vi "用户注册.vi"(8 "错误输入（无错误）":errorcluster, 11 "excel路径":path) -> (0 "错误输出":errorcluster)   [LabVIEW 2014]
panel:
  in  "取消注册":bool
  in  "注册":bool
  in  "入学年份:":string[][](array[string])
  in  "修读专业:":string[][](array[string])
  in  "修读学院:":string[][](array[string])
  in  "生日：":string[][](array[string])
  in  "民族：":string[][](array[string])
  in  "性别：":string[][](array[string])
  in  "学生姓名：":string[][](array[string])
  in  "学号：":string[][](array[string])
  # "用户注册界面"
  # "基本信息"
  # "（必填）"
  # "（必填）"
  # "学习信息"
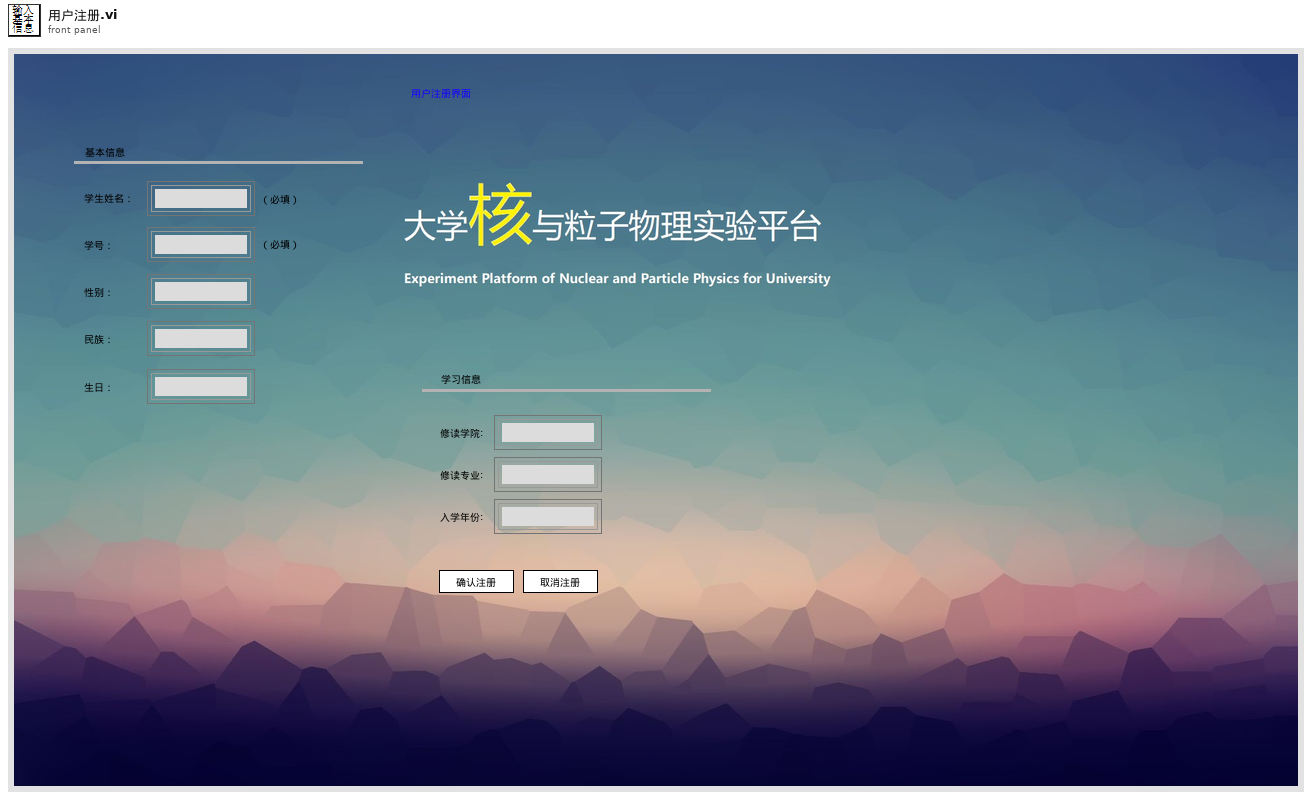
[diagram p1: front panel]
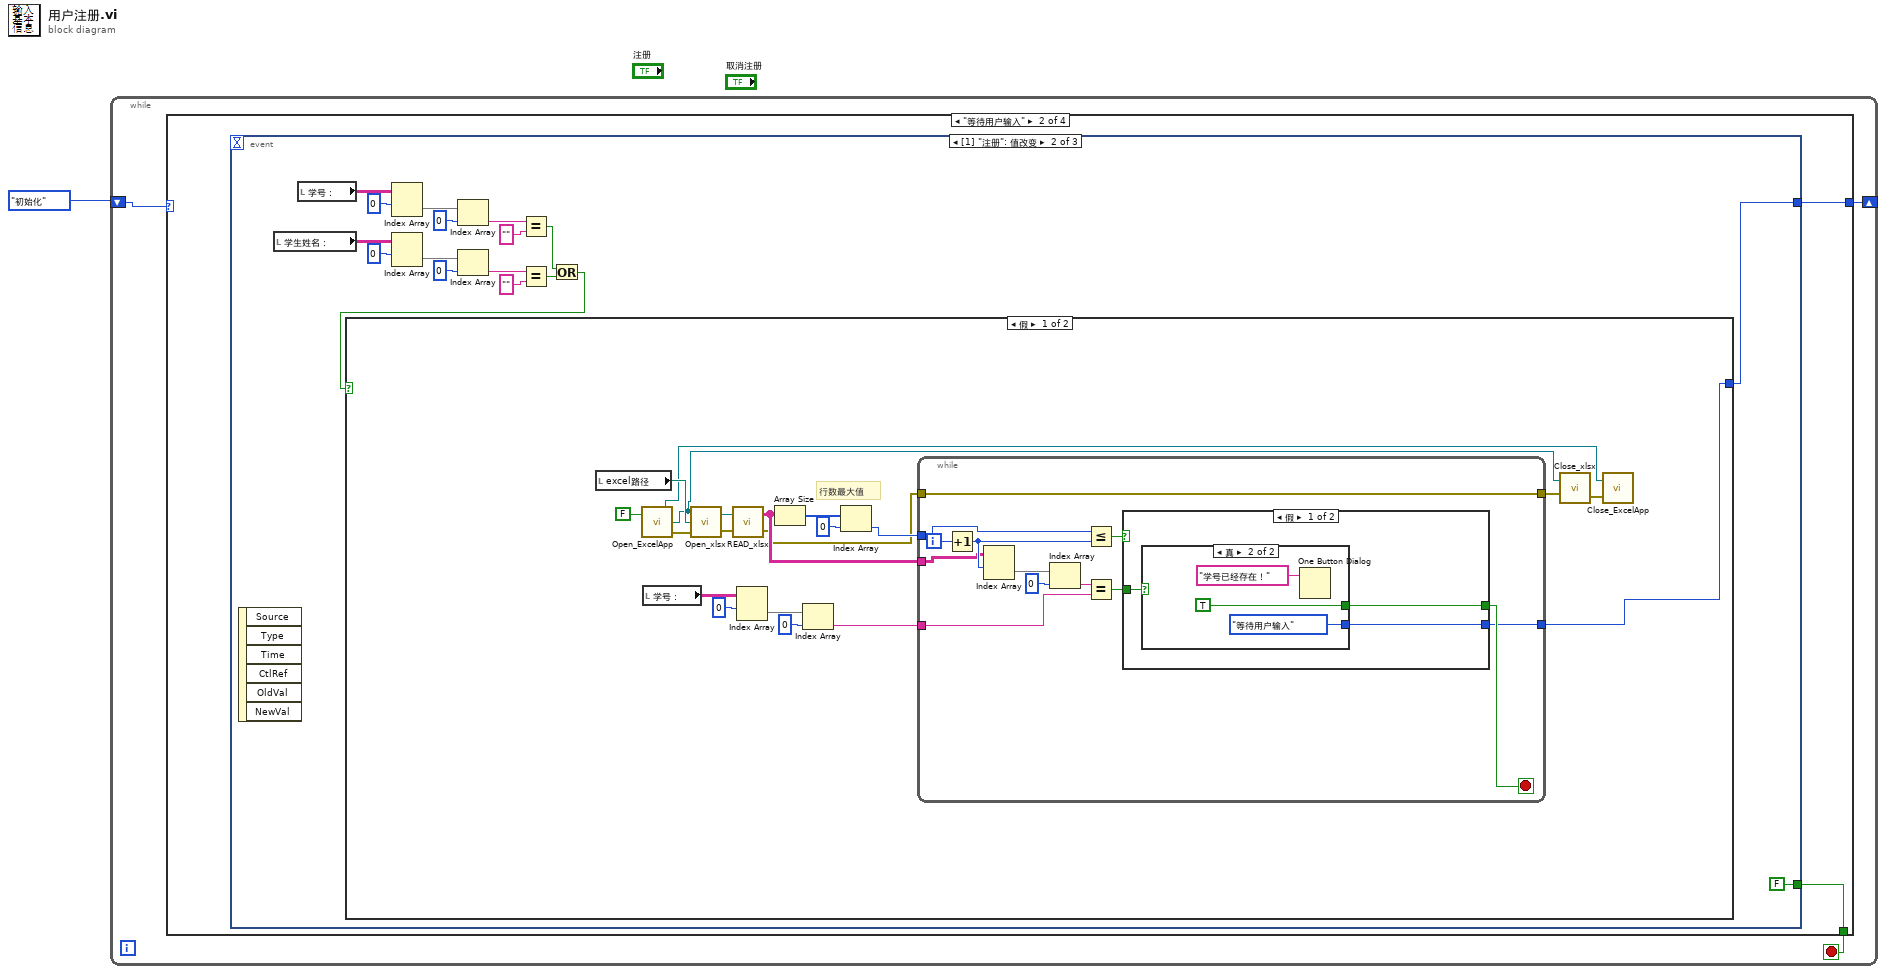
[diagram p0: block diagram]
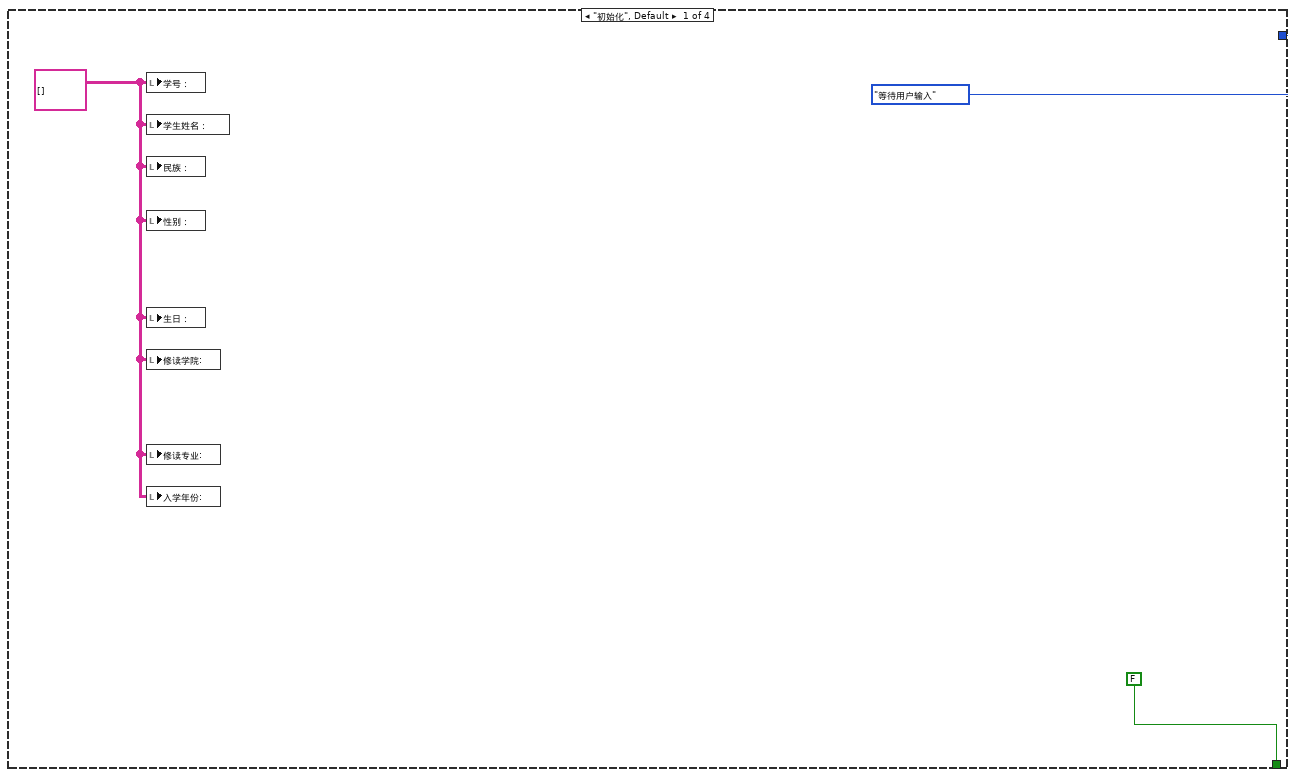
[diagram p2: hidden frame]
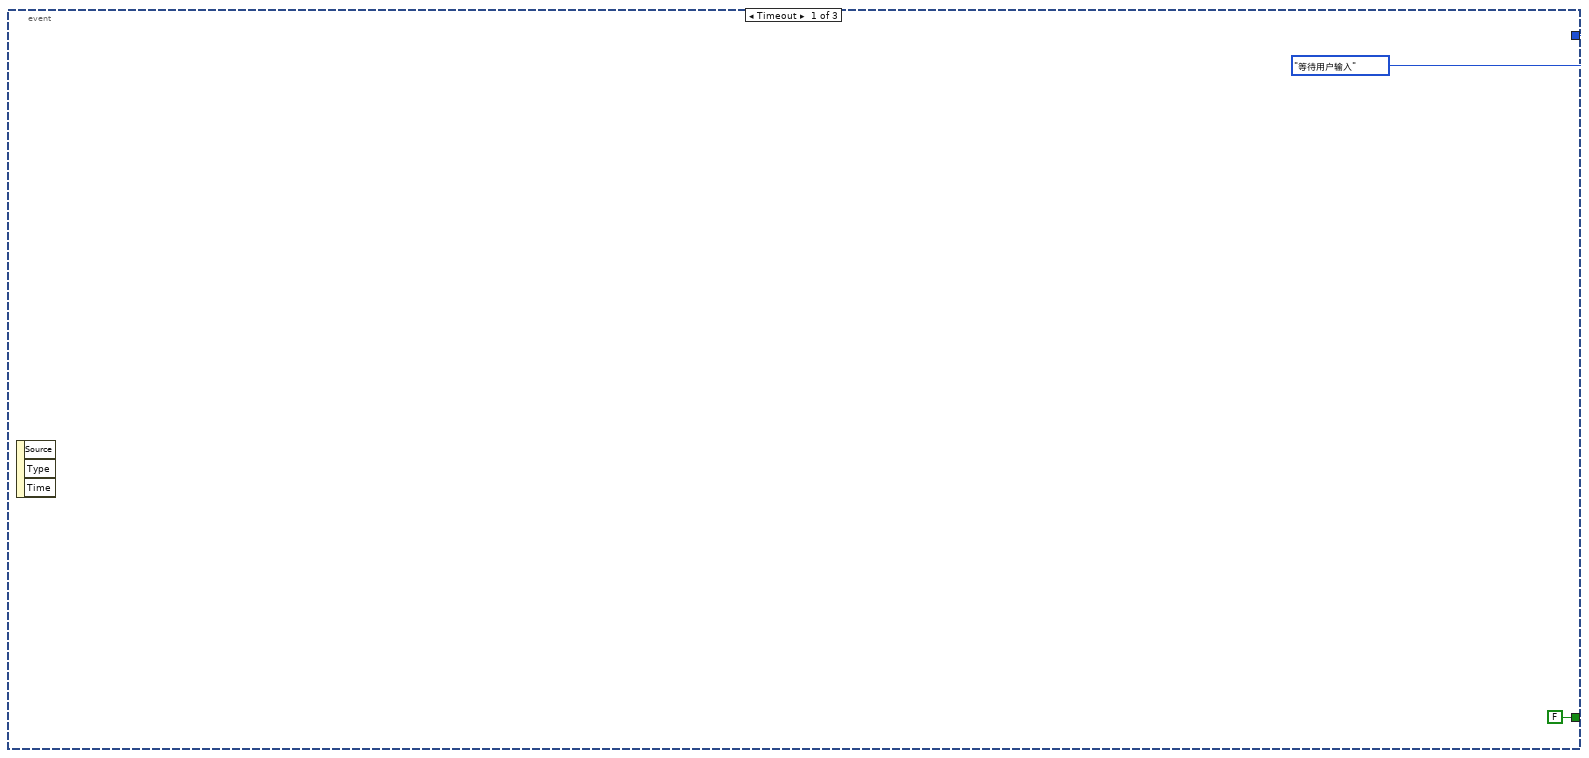
[diagram p3: hidden frame]
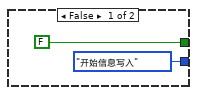
[diagram p4: hidden frame]
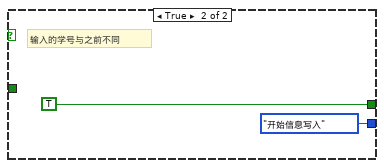
[diagram p5: hidden frame]
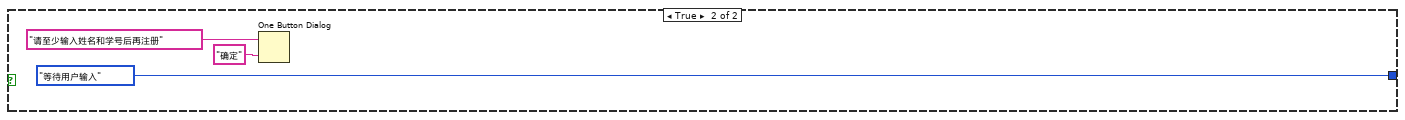
[diagram p6: hidden frame]
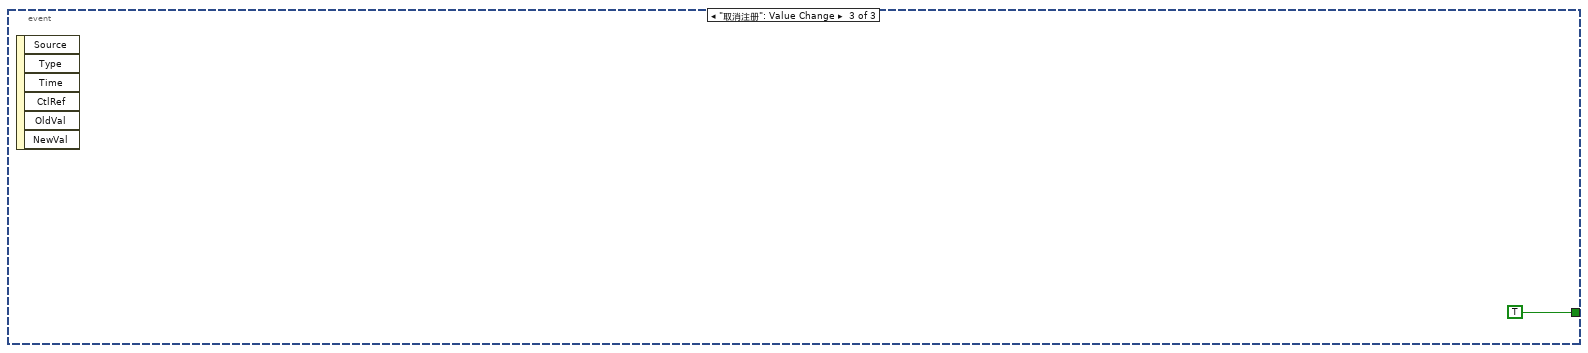
[diagram p7: hidden frame]
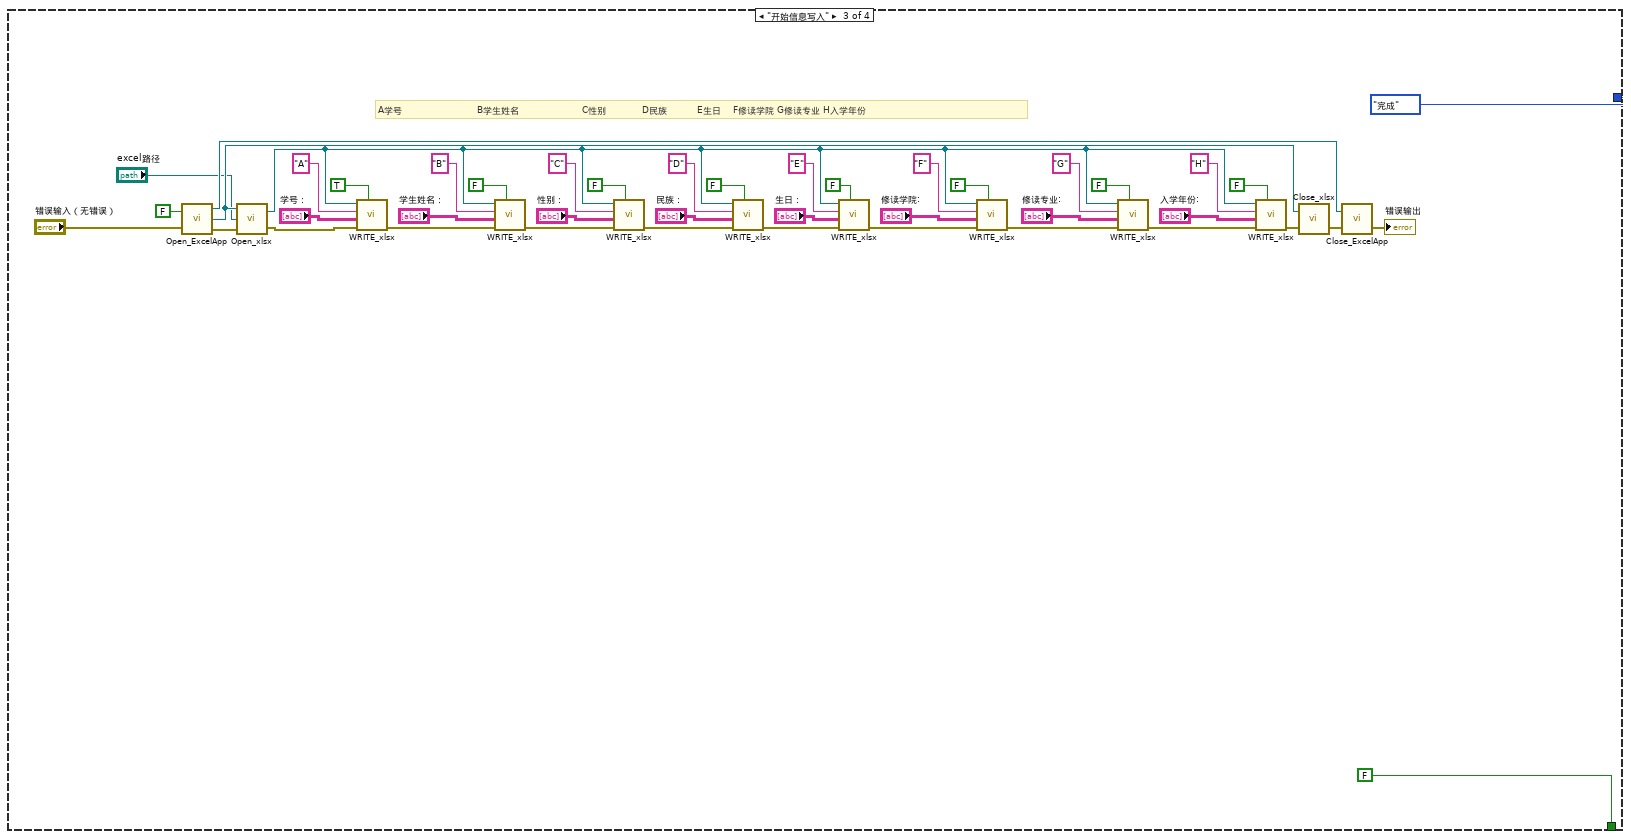
[diagram p8: hidden frame]
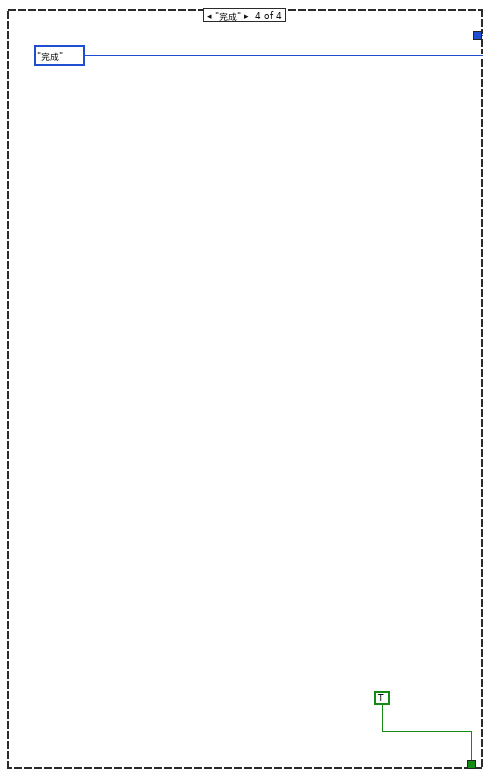
[diagram p9: hidden frame]
diagram:
  n1 = while {
    shift-right: [w2] -> _
    shift-left: enum16{"初始化", "等待用户输入", "开始信息写入", "完成"}."初始化" -> [w3]
    stop <- w4 stop-if-true
    n2 = case shown="\"等待用户输入\"" w3 {
      tunnel: [FALSE w8 FALSE TRUE] -> w4
      tunnel: [enum16{"初始化", "等待用户输入", "开始信息写入", "完成"}."等待用户输入" w9 enum16{"初始化", "等待用户输入", "开始信息写入", "完成"}."完成" enum16{"初始化", "等待用户输入", "开始信息写入", "完成"}."完成"] -> w2
      frame "初始化", Default {
        w5 = string[][] [] ("学号：")
        n3 = local write "学号："(w5) -> ()
        n4 = local write "学生姓名："(w5) -> ()
        n5 = local write "民族："(w5) -> ()
        n6 = local write "性别："(w5) -> ()
        n7 = local write "生日："(w5) -> ()
        n8 = local write "修读学院:"(w5) -> ()
        n9 = local write "修读专业:"(w5) -> ()
        n10 = local write "入学年份:"(w5) -> ()
      }
      frame "等待用户输入" {
        n11 = event shown="[1] \"注册\": 值改变" {
          selector: _ -> [_ _ _]
          dyn-events: _ -> [_ _ _]
          timeout: _ -> [_ _ _]
          tunnel: [enum16{"初始化", "等待用户输入", "开始信息写入", "完成"}."等待用户输入" w13 _] -> w9
          tunnel: [FALSE FALSE TRUE] -> w8
          event Timeout {
            n12 = event-data() -> ()  [unwired: 1 in, 3 out]
          }
          event "注册": Value Change {
            n13 = event-data() -> ()  [unwired: 1 in, 6 out]
            n14 = local read "学生姓名："() -> (w17:string[][])
            n15 = local read "学号："() -> (w28:string[][])
            n16 = Index Array(array=w28, index (row)=0 ("索引 (行)")) -> (element=w25:string[])  [unwired: 1 in]
            n17 = Index Array(array=w17, index (row)=0 ("索引 (行)")) -> (element=w20:string[])  [unwired: 1 in]
            n18 = Index Array(array=w25, index=0 ("索引 (行)")) -> (element=w24:string)
            n19 = Index Array(array=w20, index=0 ("索引 (行)")) -> (element=w21:string)
            n20 = Equal?(x=w24, y="") -> (x = y?=w16:bool)
            n21 = Equal?(x=w21, y="") -> (x = y?=w15:bool)
            n22 = Or(x=w16, y=w15) -> (x .or. y?=w14:bool)
            n23 = case shown="假" w14 {
              tunnel: [w48 enum16{"初始化", "等待用户输入", "开始信息写入", "完成"}."等待用户输入"] -> w13
              frame False {
                # "行数最大值"
                n24 = local read "excel路径"() -> (w41:path)
                n25 = call "Open_ExcelApp.vi"("excel是否可见"=FALSE) -> ("application引用"=w31:refnum<k7>, "documentl引用"=w32:refnum<k7>, "错误输出"=w37:errorcluster)  [unwired: 1 in]
                n26 = local read "学号："() -> (w46:string[][])
                n27 = call "Open_xlsx.vi"("错误输入（无错误）"=w37, "excel路径"=w41, "document引用"=w32) -> ("错误输出"=w39:errorcluster, "该文档引用输出"=w40:refnum<k7>)
                n28 = call "READ_xlsx.vi"("错误输入（无错误）"=w39, "该文档引用输入"=w40) -> ("错误输出"=w30:errorcluster, "文档内容输出"=w42:string[][])
                n29 = Index Array(array=w46, index (row)=0 ("索引 (行)")) -> (element=w43:string[])  [unwired: 1 in]
                n30 = Array Size(array=w42) -> (size(s)=w34:i32[])
                n31 = Index Array(array=w43, index=0 ("索引 (行)")) -> (element=w47:string)
                n32 = Index Array(array=w34, index=0 ("索引")) -> (element=w36:i32)
                n33 = while {
                  tunnel: w36 -> [w58]
                  tunnel: w42 -> [w57]
                  tunnel: w47 -> [w55]
                  tunnel: [w50] -> w48
                  tunnel: w30 -> [w49]
                  tunnel: [w49] -> w29
                  i -> [w59]
                  stop <- w52 stop-if-true
                  n34 = Increment(x=w59) -> (x+1=w60:i32)
                  n35 = Index Array(array=w57, index (row)=w60) -> (element=w56:string[])  [unwired: 1 in]
                  n36 = Index Array(array=w56, index=0 ("索引")) -> (element=w54:string)
                  n37 = Less Or Equal?(x=w58, y=w60) -> (x <= y?=w53:bool)
                  n38 = Equal?(x=w54, y=w55) -> (x = y?=w51:bool)
                  n39 = case shown="假" w53 {
                    tunnel: [w63 TRUE] -> w52
                    tunnel: w51 -> [w64 _]
                    tunnel: [w62 enum16{"初始化", "等待用户输入", "开始信息写入", "完成"}."开始信息写入"] -> w50
                    frame False {
                      n40 = case shown="真" w64 {
                        tunnel: [FALSE TRUE] -> w63
                        tunnel: [enum16{"初始化", "等待用户输入", "开始信息写入", "完成"}."开始信息写入" enum16{"初始化", "等待用户输入", "开始信息写入", "完成"}."等待用户输入"] -> w62
                        frame False {
                        }
                        frame True {
                          n41 = One Button Dialog(message="学号已经存在！" ("消息")) -> ()  [unwired: 1 in, 1 out]
                        }
                      }
                    }
                    frame True {
                      # "输入的学号与之前不同"
                    }
                  }
                }
                n42 = call "Close_xlsx.vi"("错误输入（无错误）"=w29, "document引用"=w32) -> ("错误输出"=w33:errorcluster)  [unwired: 1 in]
                n43 = call "Close_ExcelApp.vi"("错误输入（无错误）"=w33, "application引用"=w31) -> ()  [unwired: 1 in, 1 out]
              }
              frame True {
                n44 = One Button Dialog(message="请至少输入姓名和学号后再注册" ("消息"), button name ("OK")="确定" ("按钮名称（“确定”）")) -> ()  [unwired: 1 out]
              }
            }
          }
          event "取消注册": Value Change {
            n45 = event-data() -> ()  [unwired: 1 in, 6 out]
          }
        }
      }
      frame "开始信息写入" {
        # "A学号                         B学生姓名                     C性别            D民族          E生日    F修读学院 G修读专业 H入学年份"
        n46 = call "Open_ExcelApp.vi"("excel是否可见"=FALSE, "错误输入（无错误）"="错误输入（无错误）") -> ("application引用"=w115:refnum<k7>, "documentl引用"=w112:refnum<k7>, "错误输出"=w79:errorcluster)
        n47 = call "Open_xlsx.vi"("错误输入（无错误）"=w79, "excel路径"="excel路径", "document引用"=w112) -> ("错误输出"=w81:errorcluster, "该文档引用输出"=w111:refnum<k7>)
        n48 = call "WRITE_xlsx.vi"("是否下一行输入？"=TRUE, "错误输入（无错误）"=w81, "输入内容"="学号：", "输入列字母"="A", "该文档引用输入"=w111) -> ("错误输出"=w84:errorcluster)  [unwired: 6 in]
        n49 = call "WRITE_xlsx.vi"("是否下一行输入？"=FALSE, "错误输入（无错误）"=w84, "输入内容"="学生姓名：", "输入列字母"="B", "该文档引用输入"=w111) -> ("错误输出"=w90:errorcluster)  [unwired: 6 in]
        n50 = call "WRITE_xlsx.vi"("是否下一行输入？"=FALSE, "错误输入（无错误）"=w90, "输入内容"="性别：", "输入列字母"="C", "该文档引用输入"=w111) -> ("错误输出"=w94:errorcluster)  [unwired: 6 in]
        n51 = call "WRITE_xlsx.vi"("是否下一行输入？"=FALSE, "错误输入（无错误）"=w94, "输入内容"="民族：", "输入列字母"="D", "该文档引用输入"=w111) -> ("错误输出"=w98:errorcluster)  [unwired: 6 in]
        n52 = call "WRITE_xlsx.vi"("是否下一行输入？"=FALSE, "错误输入（无错误）"=w98, "输入内容"="生日：", "输入列字母"="E", "该文档引用输入"=w111) -> ("错误输出"=w102:errorcluster)  [unwired: 6 in]
        n53 = call "WRITE_xlsx.vi"("是否下一行输入？"=FALSE, "错误输入（无错误）"=w102, "输入内容"="修读学院:", "输入列字母"="F", "该文档引用输入"=w111) -> ("错误输出"=w106:errorcluster)  [unwired: 6 in]
        n54 = call "WRITE_xlsx.vi"("是否下一行输入？"=FALSE, "错误输入（无错误）"=w106, "输入内容"="修读专业:", "输入列字母"="G", "该文档引用输入"=w111) -> ("错误输出"=w110:errorcluster)  [unwired: 6 in]
        n55 = call "WRITE_xlsx.vi"("是否下一行输入？"=FALSE, "错误输入（无错误）"=w110, "输入内容"="入学年份:", "输入列字母"="H", "该文档引用输入"=w111) -> ("错误输出"=w113:errorcluster)  [unwired: 6 in]
        n56 = call "Close_xlsx.vi"("错误输入（无错误）"=w113, "document引用"=w112) -> ("错误输出"=w114:errorcluster)  [unwired: 1 in]
        n57 = call "Close_ExcelApp.vi"("错误输入（无错误）"=w114, "application引用"=w115) -> ("错误输出"=→"错误输出":errorcluster)  [unwired: 1 in]
      }
      frame "完成" {
      }
    }
  }
